vi "ADS1115_FT232H_Init_I2C.vi"(0 "Config":T1={"ClockRate"=100000, "LatencyTimer"=1, "Disable 3 phase clocking"=FALSE, "Disable drive only 0"=FALSE} {"ClockRate" items=["I2C_CLOCK_STANDARD_MODE"=100000, "I2C_CLOCK_FAST_MODE"=400000, "I2C_CLOCK_FAST_MODE_PLUS"=1000000, "I2C_CLOCK_HIGH_SPEED_MODE"=3400000]}) -> (14 "handle out":u32, 16 "Serial number":string, 17 "Description":string, 19 "error out":errorcluster)   [LabVIEW 2017]
uses:
  libMPSSE.lvlib
panel:
  out "numChannels out":u32
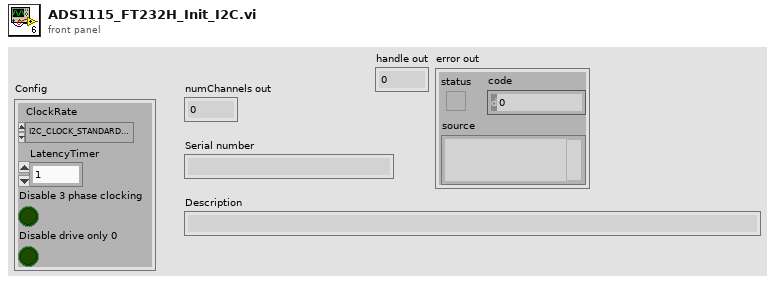
[diagram p1: front panel]
types:
  T1 = cluster{"ClockRate":u32, "LatencyTimer":u8, "Disable 3 phase clocking":bool, "Disable drive only 0":bool}
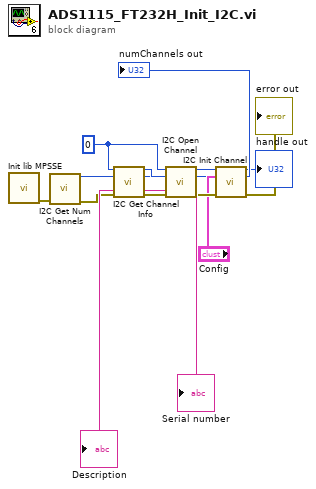
[diagram p0: block diagram]
diagram:
  w7 = u32 0 ("index")
  n1 = call "Init lib MPSSE.vi"() -> ("error out"=w3:errorcluster)  [unwired: 15 in]
  n2 = call "I2C Get Num Channels.vi"("error in (no error)"=w3) -> ("numChannels out"=→"numChannels out":u32, "error out"=w5:errorcluster)  [unwired: 13 in]
  n3 = call "I2C Get Channel Info.vi"("index"=w7, "error in (no error)"=w5) -> ("ftHandle"=w11:u32, "Description"=→"Description":string, "Serial number"=→"Serial number":string, "error out"=w6:errorcluster)  [unwired: 6 in, 4 out]
  n4 = call "I2C Open Channel.vi"("handle"=w7, "index"=w11, "error in (no error)"=w6) -> ("handle out"=w9:u32, "error out"=w10:errorcluster)  [unwired: 11 in]
  n5 = call "I2C Init Channel.vi"("handle"=w9, "Config"="Config", "error in (no error)"=w10) -> ("handle out"=→"handle out":u32, "error out"=→"error out":errorcluster)  [unwired: 11 in]
